vi "setFreqVI.vi"(1 "error in":errorcluster, 2 "Frequenz in Hz":dbl) -> (0 "error out":errorcluster)   [LabVIEW 2010]
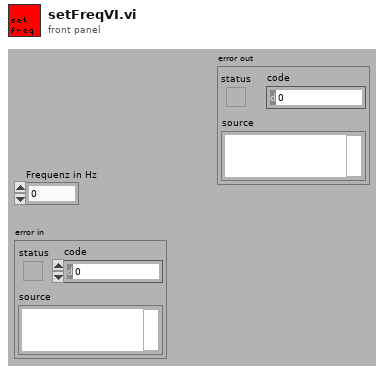
[diagram p1: front panel]
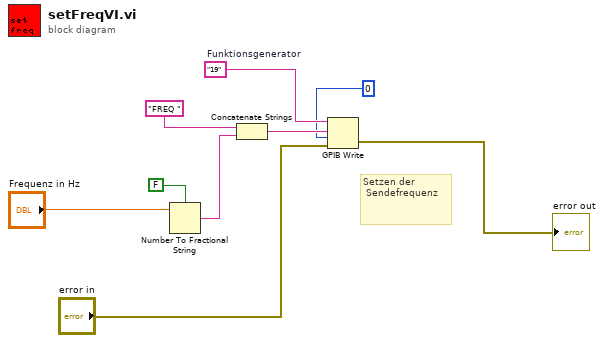
[diagram p0: block diagram]
diagram:
  w4 = "19"  # Funktionsgenerator
  # "Setzen der \n Sendefrequenz"
  n1 = Number To Fractional String(use system decimal point (T)=FALSE, number="Frequenz in Hz") -> (F-format string=w7:string)  [unwired: 2 in]
  n2 = Concatenate Strings("FREQ ", w7) -> (w5:string)
  n3 = GPIB Write(0:w4, 1:w5, 2:i16 0 ("mode (0)"), 3:"error in") -> (6:→"error out":errorcluster)  [unwired: 1 in, 1 out]
